vi "GlobalVariables.vi"() -> ()   [LabVIEW 2025, in "MySMU.lvlib"]
uses:
  MySMU.lvlib
panel:
  in  "Error Query":bool=TRUE
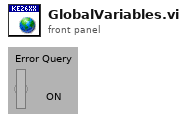
[diagram p1: front panel]
diagram:
